vi "Release Context.vi"(8 "error in":errorcluster) -> (0 "error out":errorcluster, 3 "context":refnum<class "zmq_context.lvclass">)   [LabVIEW 2019, in "RemoteControl.ZMQ.lvlib" / "ZMQ.ContextManager.lvlib"]
uses:
  ZMQ.ContextManager.lvlib
  <vilib>/addons/zeromq/zmq_context.lvclass
  Typedefs/Action--enum.ctl
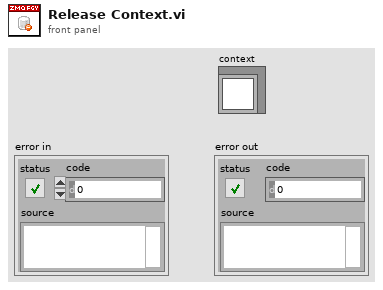
[diagram p1: front panel]
types:
  T1 = typedef "RemoteControl.ZMQ.lvlib/ZMQ.ContextManager.lvlib/Action--enum.ctl" = enum16{"Get Context", "Release Context", "Force Cleanup"}
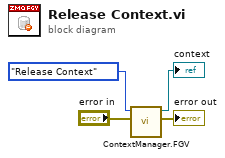
[diagram p0: block diagram]
diagram:
  n1 = call "ContextManager.FGV.vi"("error in"="error in", "action"=Action--enum."Release Context") -> ("error out"=→"error out":errorcluster, "context"=→"context":refnum<class "zmq_context.lvclass">)  [unwired: 8 in]
